vi "_PC_Pub array_most_value.vi"(0 "Array":dbl[](array[numeric])) -> (1 "sorted array":dbl[](array[numeric]), 2 "appended array":dbl[](array[numeric]))   [LabVIEW 2018]
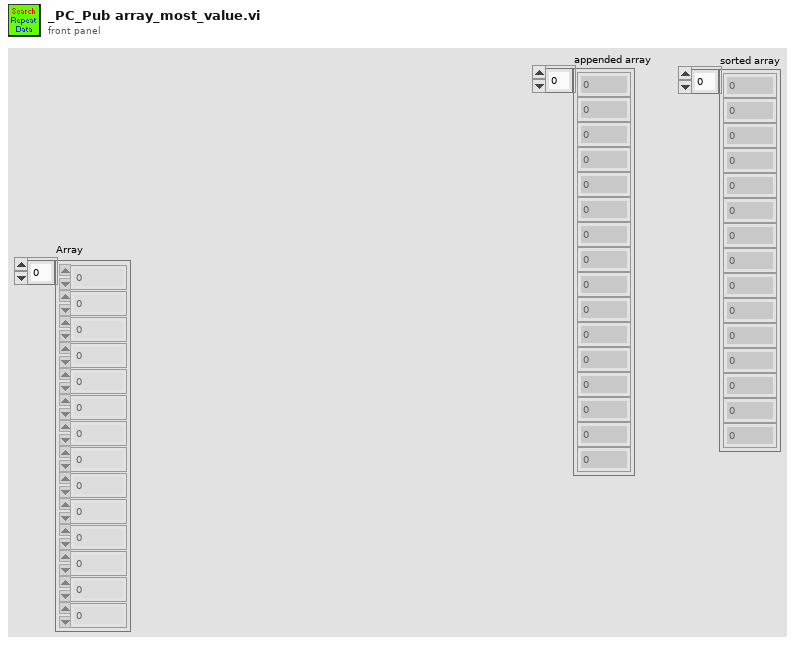
[diagram p1: front panel]
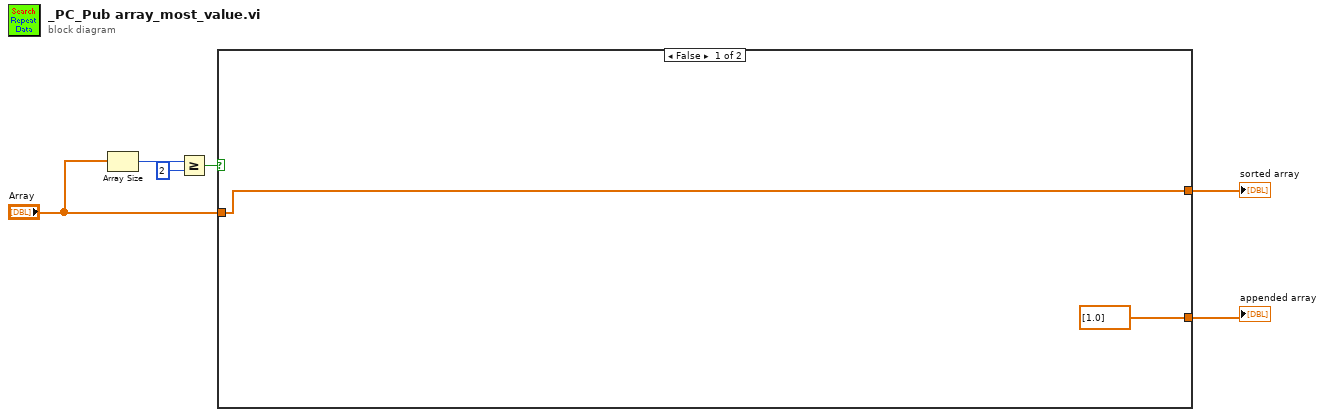
[diagram p0: block diagram]
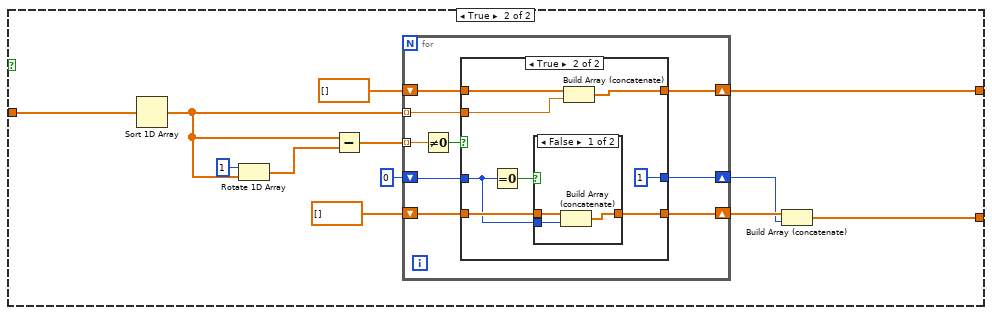
[diagram p2: hidden frame]
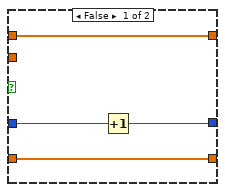
[diagram p3: hidden frame]
diagram:
  n1 = Array Size(array="Array") -> (size(s)=w5:i32)
  n2 = Greater Or Equal?(x=w5, y=2) -> (x >= y?=w3:bool)
  n3 = case shown="False" w3 {
    tunnel: "Array" -> [w8 w11]
    tunnel: [dbl[] [1.0] w10] -> w2
    tunnel: [w8 w9] -> w1
    frame False {
    }
    frame True {
      n4 = Sort 1D Array(array=w11) -> (sorted array=w17:dbl[])
      n5 = Rotate 1D Array(1:w17, 2:1 ("n")) -> (0:w19:dbl[])
      n6 = Subtract(x=w17, y=w19) -> (x-y=w18:dbl[])
      n7 = for {
        tunnel: w18 -> [w29] mode=indexing
        tunnel: w17 -> [w27] mode=indexing
        shift-right: [w25] -> w9
        shift-left: dbl[] [] ("sorted array") -> [w26]
        shift-right: [w24] -> w12
        shift-left: 0 -> [w23]
        shift-right: [w21] -> w13
        shift-left: dbl[] [] ("sorted array") -> [w22]
        n8 = Not Equal To 0?(x=w29) -> (x != 0?=w28:bool)
        n9 = case shown="True" w28 {
          tunnel: w27 -> [_ w40]
          tunnel: w26 -> [w33 w41]
          tunnel: [w33 w39] -> w25
          tunnel: [w31 1] -> w24
          tunnel: w23 -> [w32 w35]
          tunnel: w22 -> [w30 w36]
          tunnel: [w30 w34] -> w21
          frame False {
            n10 = Increment(x=w32) -> (x+1=w31:i32)
          }
          frame True {
            n11 = Equal To 0?(x=w35) -> (x = 0?=w37:bool)
            n12 = case shown="False" w37 {
              tunnel: w36 -> [w44 w45]
              tunnel: w35 -> [w43 _]
              tunnel: [w42 w45] -> w34
              frame False {
                n13 = Build Array (concatenate)(w44, w43) -> (w42:dbl[])
              }
              frame True {
              }
            }
            n14 = Build Array (concatenate)(w41, w40) -> (w39:dbl[])
          }
        }
      }
      n15 = Build Array (concatenate)(w13, w12) -> (w10:dbl[])
    }
  }
  "appended array" <- w2
  "sorted array" <- w1
